vi "lv_mysql_conn_length_coded_binary.vi"(2 "Start Index":i32, 3 "Data":u8[](array[numeric])) -> (0 "Next Index":i32, 1 "Output":u64)   [LabVIEW 2020]
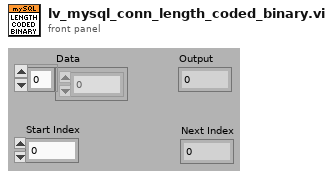
[diagram p1: front panel]
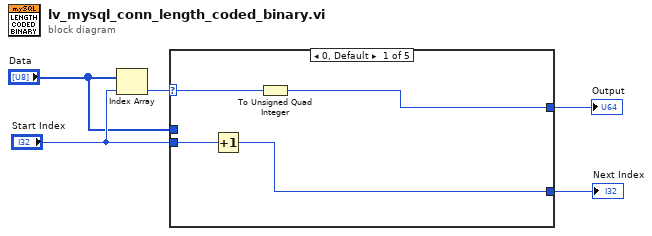
[diagram p0: block diagram]
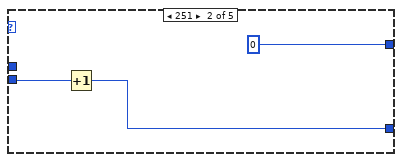
[diagram p2: hidden frame]
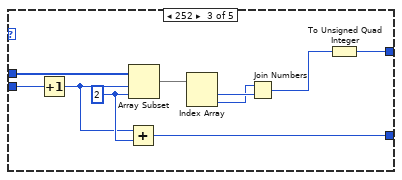
[diagram p3: hidden frame]
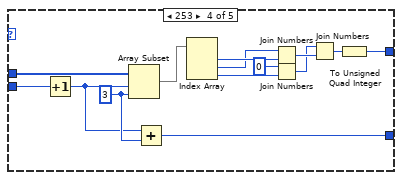
[diagram p4: hidden frame]
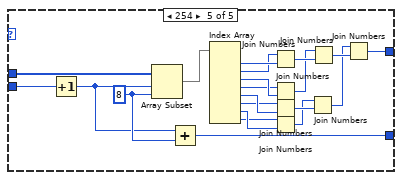
[diagram p5: hidden frame]
diagram:
  n1 = Index Array(array="Data", index="Start Index") -> (element=w2:u8)
  n2 = case shown="0, Default" w2 {
    selector: w2 -> [w9 _ _ _ _]
    tunnel: [w8 u64 0 w16 w26 w42] -> w3
    tunnel: "Data" -> [_ _ w22 w36 w40]
    tunnel: "Start Index" -> [w7 w11 w14 w28 w38]
    tunnel: [w6 w10 w18 w29 w41] -> w1
    frame 0, Default {
      n3 = Increment(x=w7) -> (x+1=w6:i32)
      n4 = To Unsigned Quad Integer(1:w9) -> (0:w8:u64)
    }
    frame 251 {
      n5 = Increment(x=w11) -> (x+1=w10:i32)
    }
    frame 252 {
      w15 = 2 ("length")
      n6 = Increment(x=w14) -> (x+1=w13:i32)
      n7 = Add(x=w13, y=w15) -> (x+y=w18:i32)
      n8 = Array Subset(array=w22, index=w13, length=w15) -> (w21:u8[])
      n9 = Index Array(array=w21) -> (element #1=w20:u8, element #2=w19:u8)  [unwired: 2 in]
      n10 = Join Numbers(hi=w19, lo=w20) -> ((hi.lo)=w17:u16)
      n11 = To Unsigned Quad Integer(1:w17) -> (0:w16:u64)
    }
    frame 253 {
      w25 = 3 ("length")
      n12 = Increment(x=w28) -> (x+1=w24:i32)
      n13 = Array Subset(array=w36, index=w24, length=w25) -> (w35:u8[])
      n14 = Add(x=w24, y=w25) -> (x+y=w29:i32)
      n15 = Index Array(array=w35) -> (element #1=w34:u8, element #2=w33:u8, element #3=w31:u8)  [unwired: 3 in]
      n16 = Join Numbers(hi=w33, lo=w34) -> ((hi.lo)=w32:u16)
      n17 = Join Numbers(hi=u8 0, lo=w31) -> ((hi.lo)=w30:u16)
      n18 = Join Numbers(hi=w30, lo=w32) -> ((hi.lo)=w27:u32)
      n19 = To Unsigned Quad Integer(1:w27) -> (0:w26:u64)
    }
    frame 254 {
      w39 = 8 ("y")
      n20 = Increment(x=w38) -> (x+1=w37:i32)
      n21 = Array Subset(array=w40, index=w37, length=w39) -> (w57:u8[])
      n22 = Add(x=w37, y=w39) -> (x+y=w41:i32)
      n23 = Index Array(array=w57) -> (element #1=w56:u8, element #2=w55:u8, element #3=w53:u8, element #4=w52:u8, element #5=w50:u8, element #6=w49:u8, element #7=w48:u8, element #8=w47:u8)  [unwired: 8 in]
      n24 = Join Numbers(hi=w55, lo=w56) -> ((hi.lo)=w54:u16)
      n25 = Join Numbers(hi=w52, lo=w53) -> ((hi.lo)=w51:u16)
      n26 = Join Numbers(hi=w49, lo=w50) -> ((hi.lo)=w46:u16)
      n27 = Join Numbers(hi=w47, lo=w48) -> ((hi.lo)=w45:u16)
      n28 = Join Numbers(hi=w45, lo=w46) -> ((hi.lo)=w43:u32)
      n29 = Join Numbers(hi=w51, lo=w54) -> ((hi.lo)=w44:u32)
      n30 = Join Numbers(hi=w43, lo=w44) -> ((hi.lo)=w42:u64)
    }
  }
  "Output" <- w3
  "Next Index" <- w1
